vi "case_pause_torture.vi"(7 "Main VI reference":refnum<vi>, 8 "error in (no error)":errorcluster, 9 "queue in":refnum<queue>, 11 "VISA resource name in":refnum<visa-resource-name>) -> (0 "error out":errorcluster, 3 "VISA Refnum out":refnum<visa-resource-name>)   [LabVIEW 2020]
uses:
  controls/message cluster.ctl
  <instrlib>/Marlin Instrument Driver/Public/controls/move parameters.ctl
  0d3c9508-d22d-4d7f-953c-a106fea8de4a.vi
  <instrlib>/Marlin Instrument Driver/Marlin Instrument Driver.lvlib
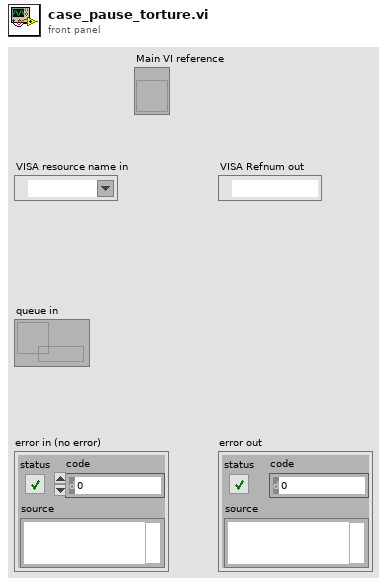
[diagram p1: front panel]
types:
  T1 = typedef "Marlin Instrument Driver.lvlib/move parameters.ctl" = cluster{"E":dbl, "F":dbl, "X":dbl, "Y":dbl, "Z":dbl}
  T2 = typedef "message cluster.ctl" = cluster{"message":string, "data":variant}
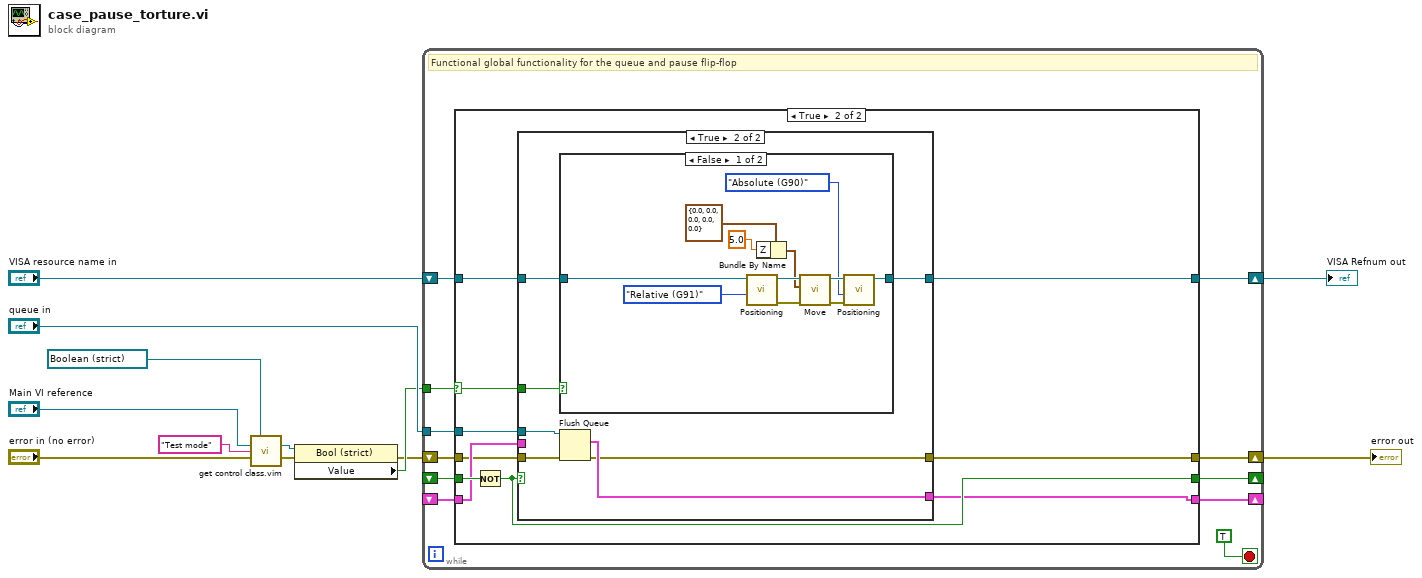
[diagram p0: block diagram]
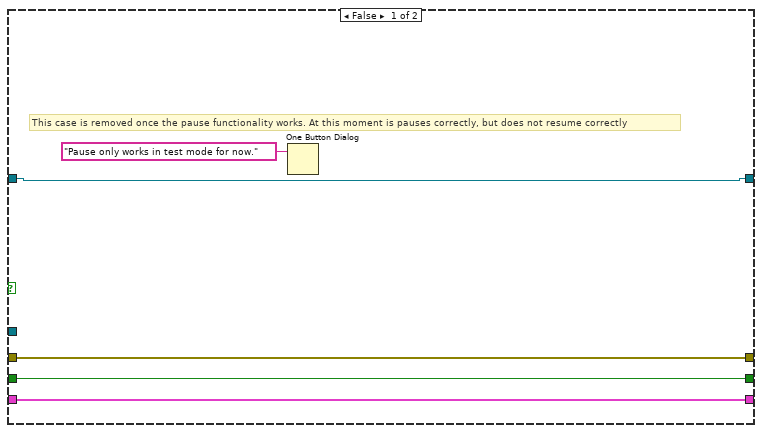
[diagram p2: hidden frame]
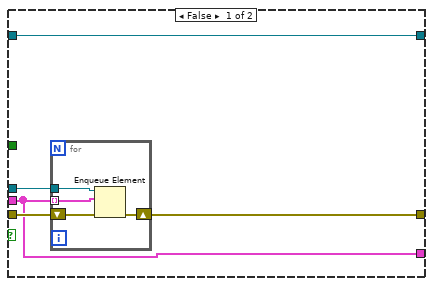
[diagram p3: hidden frame]
diagram:
  n1 = call "get control class.vim"("Control class"=refnum<vi> refnum ("Test mode"), "Main VI reference"="Main VI reference", "Label"="Test mode", "error in (no error)"="error in (no error)") -> ("Control out"=w7:refnum<vi>, "error out"=w6:errorcluster)  [unwired: 10 in]
  n2 = property on="Property Node" class="Bool (strict)"(reference=w7, error in=w6) -> (error out=w1:errorcluster, "Value"=w3:bool)  [unwired: 1 out]
  n3 = while {
    tunnel: "queue in" -> [w17]
    tunnel: w3 -> [w15]
    shift-right: [w23] -> w12
    shift-left: "VISA resource name in" -> [w22]
    shift-right: [w19] -> _
    shift-left: _ -> [w20]
    shift-right: [w18] -> _
    shift-left: _ -> [w16]
    shift-right: [w21] -> w10
    shift-left: w1 -> [w14]
    stop <- TRUE stop-if-true
    # "Functional global functionality for the queue and pause flip-flop"
    n4 = case shown="True" w15 {
      selector: w15 -> [_ w29]
      tunnel: w16 -> [w25 w38]
      tunnel: w17 -> [_ w37]
      tunnel: [w25 w36] -> w18
      tunnel: [w28 w35] -> w19
      tunnel: w20 -> [w28 w34]
      tunnel: w14 -> [w26 w33]
      tunnel: [w26 w32] -> w21
      tunnel: w22 -> [w27 w31]
      tunnel: [w27 w30] -> w23
      frame False {
        # "This case is removed once the pause functionality works. At this moment is pauses correctly, but does not resume correctly"
        n5 = One Button Dialog(message="Pause only works in test mode for now.") -> ()  [unwired: 1 in, 1 out]
      }
      frame True {
        n6 = Not(x=w38) -> (.not. x?=w36:bool)
        n7 = case shown="True" w36 {
          tunnel: w37 -> [w43 w54]
          tunnel: [w40 w53] -> w35
          tunnel: w34 -> [w40 _]
          tunnel: w33 -> [w42 w51]
          tunnel: [w41 w52] -> w32
          tunnel: w31 -> [w39 w50]
          tunnel: [w39 w49] -> w30
          tunnel: w29 -> [_ w48]
          frame False {
            n8 = for {
              tunnel: w43 -> [w47]
              tunnel: w40 -> [w46] mode=indexing
              shift-right: [w44] -> w41
              shift-left: w42 -> [w45]
              n9 = Enqueue Element(queue=w47, element=w46, error in (no error)=w45) -> (error out=w44:errorcluster)  [unwired: 1 in, 2 out]
            }
          }
          frame True {
            n10 = case shown="False" w48 {
              tunnel: w50 -> [w64 w66]
              tunnel: [w56 w66] -> w49
              frame False {
                n11 = call <instrlib>:"Positioning.vi"("type"=enum16{"Absolute (G90)", "Relative (G91)"}."Relative (G91)", "VISA resource name"=w64) -> ("error out"=w62:errorcluster, "VISA resource name out"=w65:refnum<visa-resource-name>)  [unwired: 8 in]
                n12 = Bundle By Name(cluster=T1 {"E"=0.0, "F"=0.0, "X"=0.0, "Y"=0.0, "Z"=0.0} ("Distances"), "Z"=5.0) -> (w57:T1)
                n13 = call <instrlib>:"Move.vi"("error in (no error)"=w62, "Distances"=w57, "VISA resource name"=w65) -> ("error out"=w61:errorcluster, "VISA resource name out"=w60:refnum<visa-resource-name>)  [unwired: 7 in]
                n14 = call <instrlib>:"Positioning.vi"("error in (no error)"=w61, "type"=enum16{"Absolute (G90)", "Relative (G91)"}."Absolute (G90)", "VISA resource name"=w60) -> ("VISA resource name out"=w56:refnum<visa-resource-name>)  [unwired: 7 in, 1 out]
              }
              frame True {
              }
            }
            n15 = Flush Queue(queue=w54, error in (no error)=w51) -> (remaining elements=w53:T2[], error out=w52:errorcluster)  [unwired: 1 out]
          }
        }
      }
    }
  }
  "VISA Refnum out" <- w12
  "error out" <- w10
